vi "GetBounds.vi"(0 "XRef":T6, 1 "State In":T4) -> (14 "Bounds":T2, 15 "Fatal Error Out":T1)   [LabVIEW 2018, in "RetryNode.xnode"]
uses:
  RetryNode.xnode
  <vilib>/XNodeSupport/XNodeXNodeRef.ctl
  State.ctl
  <vilib>/Utility/miscctls.llb/LVRectTypeDef.ctl
  <vilib>/XNodeSupport/XNodeBounds.ctl
  <vilib>/XNodeSupport/XNodeInt.ctl
  <vilib>/XNodeSupport/XNodeErrorCluster.ctl
  <vilib>/XNodeSupport/NI_XNodeSupport.lvlib
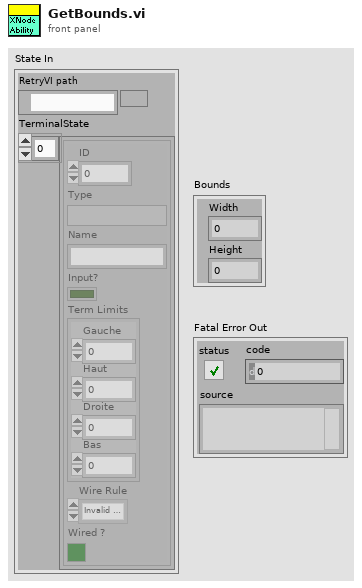
[diagram p1: front panel]
types:
  T1 = typedef "NI_XNodeSupport.lvlib/XNodeErrorCluster.ctl" = errorcluster
  T2 = typedef "NI_XNodeSupport.lvlib/XNodeBounds.ctl" = cluster{"Width":T3, "Height":T3}
  T3 = typedef "NI_XNodeSupport.lvlib/XNodeInt.ctl" = i32
  T4 = typedef "RetryNode.xnode/State.ctl" = cluster{"RetryVI path":path, "TerminalState":cluster{"ID":i32, "Type":variant, "Name":string, "Input?":bool, "Term Limits":T5, "Wire Rule":enum16{"Invalid Wire Rule", "Required", "Recommended", "Optional", "Dynamic Dispatch"}, "Wired ?":bool}[]}
  T5 = typedef "LVRectTypeDef.ctl" = cluster{"Left":i16, "Top":i16, "Right":i16, "Bottom":i16}
  T6 = typedef "NI_XNodeSupport.lvlib/XNodeXNodeRef.ctl" = refnum<vi>
  T7 = typedef "imagedata.ctl" = cluster{"image type":i32, "image depth":i32, "image":u8[], "mask":u8[], "colors":u32[], "Rectangle":cluster{"left":i16, "top":i16, "right":i16, "bottom":i16}}
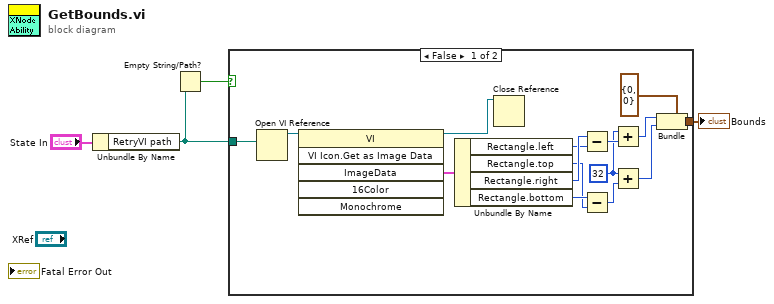
[diagram p0: block diagram]
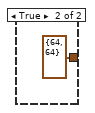
[diagram p2: hidden frame]
diagram:
  n1 = Unbundle By Name("State In") -> ("RetryVI path"=w2:path)
  n2 = Empty String/Path?(string/path=w2) -> (empty?=w1:bool)
  n3 = case shown="False" w1 {
    tunnel: [w12 T2 {"Width"=64, "Height"=64} ("Bounds")] -> w3
    tunnel: w2 -> [w6 _]
    frame False {
      w9 = 32
      n4 = Open VI Reference(vi path=w6) -> (vi reference=w19:refnum<vi>)  [unwired: 5 in, 1 out]
      n5 = invoke class="VI" method="VI Icon.Get as Image Data"(reference=w19) -> (reference out=w5:refnum<vi>, "ImageData"=w18:T7)  [unwired: 5 in, 4 out]
      n6 = Unbundle By Name(w18) -> ("Rectangle.left"=w16:i16, "Rectangle.top"=w14:i16, "Rectangle.right"=w17:i16, "Rectangle.bottom"=w15:i16)
      n7 = Close Reference(reference=w5) -> ()  [unwired: 1 in, 1 out]
      n8 = Subtract(x=w17, y=w16) -> (x-y=w11:i16)
      n9 = Subtract(x=w15, y=w14) -> (x-y=w10:i16)
      n10 = Add(x=w9, y=w11) -> (x+y=w8:i32)
      n11 = Add(x=w9, y=w10) -> (x+y=w7:i32)
      n12 = Bundle(cluster=T2 {"Width"=0, "Height"=0} ("Bounds"), "Width"=w8, "Height"=w7) -> (w12:T2)
    }
    frame True {
    }
  }
  "Bounds" <- w3
